vi "HissDemo.vi"() -> ()   [LabVIEW 2020]
panel:
  out "Numeric 2":dbl
  out "Numeric":dbl
  out "Boolean":bool
  in  "Cluster 2":T1
  out "Cluster":T2
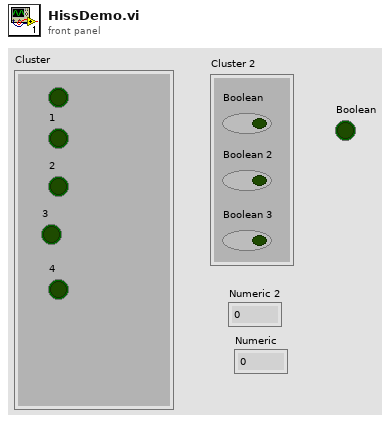
[diagram p1: front panel]
types:
  T1 = cluster{"Boolean":bool, "Boolean 2":bool, "Boolean 3":bool}
  T2 = cluster{"1":bool, "2":bool, "3":bool, "4":bool, "5":bool}
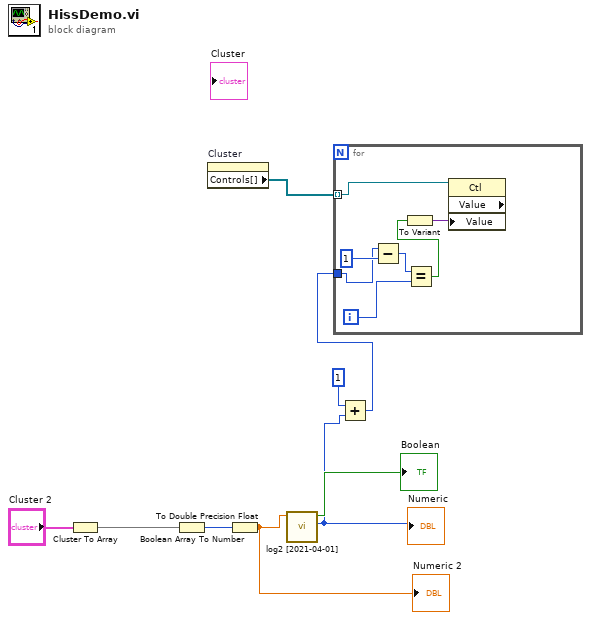
[diagram p0: block diagram]
diagram:
  n1 = Cluster To Array(cluster="Cluster 2") -> (array=w4:bool[])
  n2 = Boolean Array To Number(Boolean array=w4) -> (number=w7:u32)
  n3 = property on="Cluster" class="Clust (strict)"() -> ("Controls[]"=w9:refnum<vi>[])  [unwired: 2 in, 2 out]
  n4 = To Double Precision Float(number=w7) -> (double precision float=w5:dbl)
  "Numeric 2" <- w5
  n5 = call "log2 [2021-04-01].vi"("Input"=w5) -> ("Numeric"=w3:i32, "Boolean"=→"Boolean":bool)  [unwired: 9 in]
  "Numeric" <- w3
  n6 = Add(x=1, y=w3) -> (x+y=w1:i32)
  n7 = for {
    tunnel: w9 -> [w13] mode=indexing
    tunnel: w1 -> [w10]
    i -> [w15]
    n8 = Subtract(x=w10, y=1) -> (x-y=w14:i32)
    n9 = Equal?(x=w14, y=w15) -> (x = y?=w12:bool)
    n10 = To Variant(anything=w12) -> (Variant=w11:variant)
    n11 = property class="Ctl" props=["Value", "Value"](reference=w13, "Value"=w11) -> ()  [unwired: 1 in, 3 out]
  }
